vi "Square 00.vi"(1 "x":sgl) -> (0 "x^2":sgl)   [LabVIEW 2015]
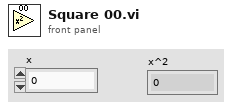
[diagram p1: front panel]
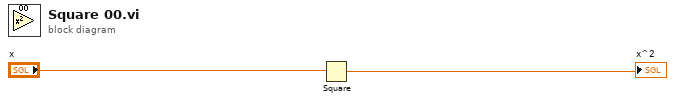
[diagram p0: block diagram]
diagram:
  n1 = Square(x="x") -> (x^2=→"x^2":sgl)
